vi "GetDevTree_LS1.vi"(8 "ErrorIn":errorcluster caption="Entrée d'erreur", 11 "TreeRefIn":refnum<vi>) -> (0 "ErrorOut":errorcluster caption="Sortie d'erreur", 3 "TreeRefOut":refnum<vi>)   [LabVIEW 2019]
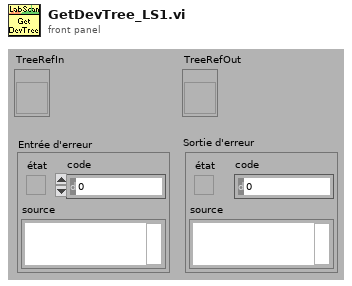
[diagram p1: front panel]
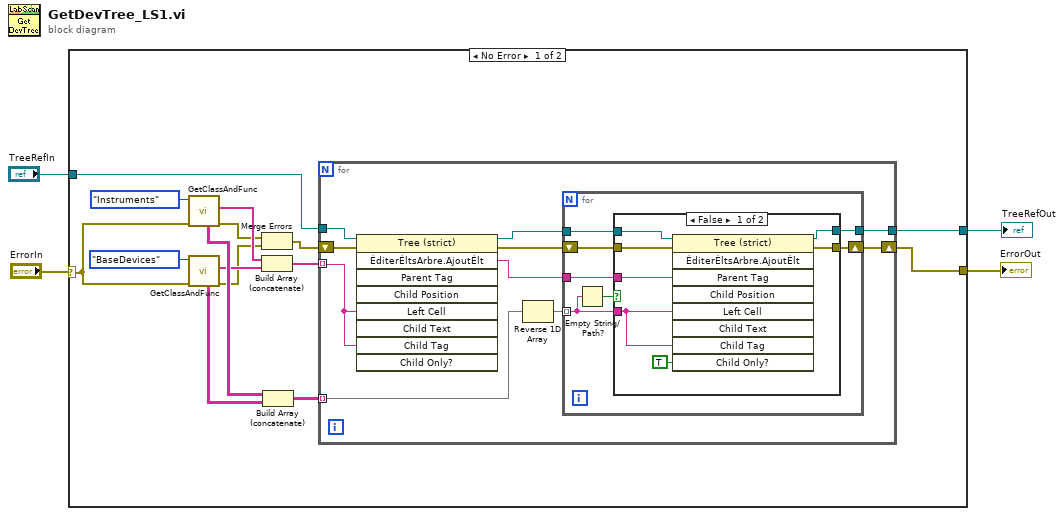
[diagram p0: block diagram]
diagram:
  n1 = case shown="No Error" "ErrorIn" {
    selector: "ErrorIn" -> [w5 w46]
    tunnel: [w11 w45] -> w4
    tunnel: [w7 w46] -> w3
    tunnel: "TreeRefIn" -> [w6 w45]
    frame No Error {
      n2 = call "GetClassAndFunc.vi"("error in (no error)"=w5, "ClassType"=enum16{"BaseDevices", "Instruments"}."Instruments") -> ("error out"=w9:errorcluster, "ClassNames"=w16:string[], "FuncNamesArr"=w18:string[][])  [unwired: 5 in, 2 out]
      n3 = call "GetClassAndFunc.vi"("error in (no error)"=w5, "ClassType"=enum16{"BaseDevices", "Instruments"}."BaseDevices") -> ("error out"=w10:errorcluster, "ClassNames"=w17:string[], "FuncNamesArr"=w19:string[][])  [unwired: 5 in, 2 out]
      n4 = Merge Errors(w9, w10) -> (w8:errorcluster)
      n5 = Build Array (concatenate)(w16, w17) -> (w12:string[])
      n6 = Build Array (concatenate)(w18, w19) -> (w13:string[][])
      n7 = for {
        tunnel: w12 -> [w29] mode=indexing
        tunnel: w13 -> [w27] mode=indexing
        shift-right: [w24] -> w7
        shift-left: w8 -> [w23]
        tunnel: w6 -> [w22]
        tunnel: [w20] -> w11
        n8 = invoke on="Nœud de méthode" class="Tree (strict)" method="ÉditerÉltsArbre.AjoutÉlt"(reference=w22, error in=w23, "Left Cell"=w29, "Child Tag"=w29) -> (reference out=w21:refnum<vi>, error out=w25:errorcluster, "Edit Tree Items:Add Item"=w28:string)  [unwired: 5 in, 6 out]
        n9 = Reverse 1D Array(array=w27) -> (reversed array=w26:string[])
        n10 = for {
          tunnel: w28 -> [w36]
          tunnel: w26 -> [w35] mode=indexing
          shift-right: [w32] -> w24
          shift-left: w25 -> [w33]
          tunnel: w21 -> [w31]
          tunnel: [w30] -> w20
          n11 = Empty String/Path?(string/path=w35) -> (empty?=w34:bool)
          n12 = case shown="False" w34 {
            tunnel: w36 -> [w43 _]
            tunnel: w35 -> [w42 _]
            tunnel: [w41 _] -> w32
            tunnel: w33 -> [w40 _]
            tunnel: w31 -> [w39 w44]
            tunnel: [w38 w44] -> w30
            frame False {
              n13 = invoke on="Nœud de méthode" class="Tree (strict)" method="ÉditerÉltsArbre.AjoutÉlt"(reference=w39, error in=w40, "Parent Tag"=w43, "Left Cell"=w42, "Child Tag"=w42, "Child Only?"=TRUE ("Enfant uniquement ?")) -> (reference out=w38:refnum<vi>, error out=w41:errorcluster)  [unwired: 3 in, 7 out]
            }
            frame True {
            }
          }
        }
      }
    }
    frame Error {
    }
  }
  "TreeRefOut" <- w4
  "ErrorOut" <- w3
